vi "Check state and switch on time.vi"(8 "error in":errorcluster, 11 "Servo Switch in":refnum<class "Servo Switch.lvclass">) -> (0 "error out":errorcluster, 1 "New Time":u32, 2 "TimeElapsed?":bool, 3 "Servo Switch out":refnum<class "Servo Switch.lvclass">, 4 "NextSwitch":dbl, 6 "LastSwitch":timestamp)   [LabVIEW 2019, in "Servo Switch.lvclass"]
doc: "Change the state of the switch and put out the new time for a switch."
uses:
  Servo Switch.lvclass
  Z:/sw_repo/handix/source/Reusable/Switch/Switch.lvclass
  Servo Switch.lvclass/Servo Switch.ctl
  Read High Time.vi
  Read Low Time.vi
  Reusable/Switch/Read maxElapsedTime.vi
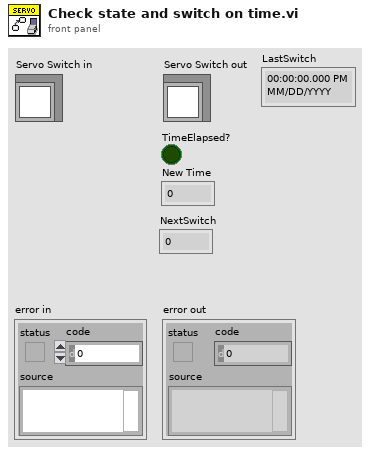
[diagram p1: front panel]
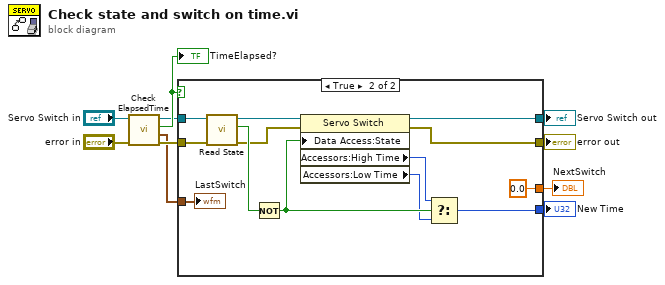
[diagram p0: block diagram]
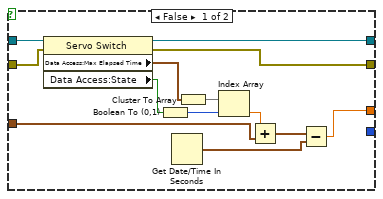
[diagram p2: hidden frame]
diagram:
  n1 = call-dynamic "Check ElapsedTime.vi"("error in"="error in", "Switch in"="Servo Switch in") -> ("error out"=w4:errorcluster, "LastSwitch"=w2:timestamp, "TimeElapsed?"=w9:bool, "Switch out"=w8:refnum<class "Servo Switch.lvclass">)  [unwired: 6 in]
  "TimeElapsed?" <- w9
  n2 = case shown="True" w9 {
    tunnel: w8 -> [w23 w30]
    tunnel: [w13 w33] -> w7
    tunnel: [_ w32] -> w6
    tunnel: w4 -> [w22 w26]
    tunnel: [w12 w31] -> w3
    tunnel: w2 -> [w16 w24]
    tunnel: [w11 0.0] -> w1
    frame False {
      n3 = property class="Servo Switch"(reference=w23, error in=w22) -> (reference out=w13:refnum<class "Servo Switch.lvclass">, error out=w12:errorcluster, "Data Access:Max Elapsed Time"=w21:cluster{"true":sgl, "false":sgl}, "Data Access:State"=w18:bool)
      n4 = Boolean To (0,1)(Boolean=w18) -> (0, 1=w17:i16)
      n5 = Get Date/Time In Seconds() -> (seconds since 1Jan1904=w14:timestamp)
      n6 = Cluster To Array(cluster=w21) -> (array=w20:sgl[])
      n7 = Index Array(array=w20, index=w17) -> (element=w19:sgl)
      n8 = Add(x=w19, y=w16) -> (x+y=w15:timestamp)
      n9 = Subtract(x=w15, y=w14) -> (x-y=w11:dbl)
    }
    frame True {
      n10 = call-dynamic "Read State.vi"("error in (no error)"=w26, "Switch in"=w30) -> ("error out"=w27:errorcluster, "State"=w28:bool, "Switch out"=w29:refnum<class "Servo Switch.lvclass">)  [unwired: 7 in]
      n11 = Not(x=w28) -> (.not. x?=w36:bool)
      n12 = property class="Servo Switch"(reference=w29, error in=w27, "Data Access:State"=w36) -> (reference out=w33:refnum<class "Servo Switch.lvclass">, error out=w31:errorcluster, "Accessors:High Time"=w35:u32, "Accessors:Low Time"=w34:u32)
      n13 = Select(t=w35, s=w36, f=w34) -> (s? t:f=w32:u32)
      "LastSwitch" <- w24
    }
  }
  "error out" <- w3
  "Servo Switch out" <- w7
  "New Time" <- w6
  "NextSwitch" <- w1
